vi "aal_Error Code Pool.vi"   [LabVIEW 2017, in "NI_AALPro.lvlib"]
uses:
  <vilib>/Analysis/NI_AALPro.lvlib
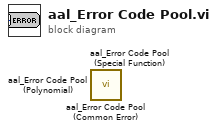
[diagram p0: block diagram]
diagram:
  n1 = call <vilib>:"aal_Error Code Pool (Common Error).vi"() -> ()  [unwired: 1 in, 1 out]
  n2 = call <vilib>:"aal_Error Code Pool (Special Function).vi"() -> ()  [unwired: 1 in, 1 out]
  n3 = call <vilib>:"aal_Error Code Pool (Polynomial).vi"() -> ()  [unwired: 1 in, 1 out]
